vi "C867_Init.vi"(8 "error in":errorcluster caption="entrée d'erreur") -> (0 "error out":errorcluster caption="sortie d'erreur", 3 "ID":i32 caption="Numérique")   [LabVIEW 2026]
uses:
  Controls/TypeDef_FGV.ctl
  C867-VIs/Low Level/PI_GCS2_DLL_x64.dll
panel:
  in  "nBaudRate":i32=115200
  in  "nPortNr":i32=15
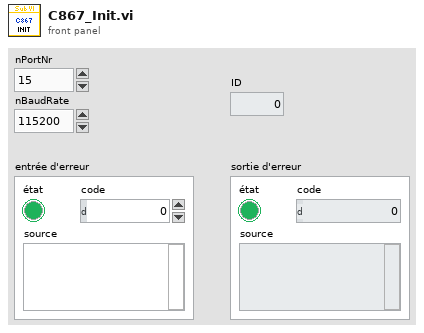
[diagram p1: front panel]
types:
  T1 = typedef "TypeDef_FGV.ctl" = enum16{"Initialize", "Write", "Read"}
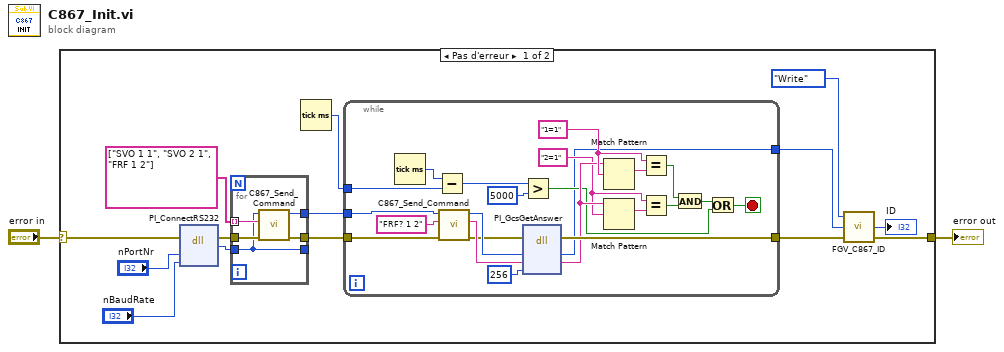
[diagram p0: block diagram]
diagram:
  n1 = case shown="Pas d'erreur" "error in" {
    selector: "error in" -> [w16 w45]
    tunnel: [w8 w45] -> w1
    frame No Error {
      n2 = dll-call lib="D:/SEBASTIEN/GitHub/LABVIEW-Useful-codes/Device_control/PC-C867-IO Control/v0.2/SubVI/PI-C867/C867-VIs/Low Level/PI_GCS2_DLL_x64.dll" fn="PI_ConnectRS232"(error in=w16, "nPortNr"="nPortNr", "nBaudRate"="nBaudRate") -> (error out=w5:errorcluster, "ID"=w6:i32)  [unwired: 4 in, 1 out]
      n3 = for {
        tunnel: string[] ["SVO 1 1", "SVO 2 1", "FRF 1 2"] -> [w18] mode=indexing
        tunnel: w5 -> [w21]
        tunnel: [w20] -> w11
        tunnel: [w17] -> _
        tunnel: [w19] -> w10
        tunnel: w6 -> [w17]
        n4 = call "C867_Send_Command.vi"("entrée d'erreur (pas d'erreur)"=w21, "szCommand"=w18, "ID en entrée"=w17) -> ("sortie d'erreur"=w20:errorcluster, "ID en sortie"=w19:i32)  [unwired: 5 in, 2 out]
      }
      n5 = Tick Count (ms)() -> (millisecond timer value=w13:u32)
      n6 = while {
        tunnel: w11 -> [w27]
        tunnel: w10 -> [w25]
        tunnel: [w44] -> w4
        tunnel: w13 -> [w41]
        tunnel: [w28] -> w3
        stop <- w31 stop-if-true
        w34 = "2=1" ("chaîne recherchée")
        w38 = "1=1" ("chaîne recherchée")
        n7 = Tick Count (ms)() -> (millisecond timer value=w42:u32)
        n8 = Subtract(x=w42, y=w41) -> (x-y=w40:u32)
        n9 = call "C867_Send_Command.vi"("entrée d'erreur (pas d'erreur)"=w27, "szCommand"="FRF? 1 2", "ID en entrée"=w25) -> ("sortie d'erreur"=w22:errorcluster, "szCommand out"=w24:string, "ID en sortie"=w23:i32)  [unwired: 5 in, 1 out]
        n10 = Greater?(x=w40, y=u32 5000) -> (0:w32:bool)
        n11 = dll-call lib="D:/SEBASTIEN/GitHub/LABVIEW-Useful-codes/Device_control/PC-C867-IO Control/v0.2/SubVI/PI-C867/C867-VIs/Low Level/PI_GCS2_DLL_x64.dll" fn="PI_GcsGetAnswer"(error in=w22, "ID"=w23, "buffer"=w24, "buffersize"=256) -> (error out=w44:errorcluster, "ID"=w28:i32, "buffer"=w36:string)  [unwired: 4 in, 1 out]
        n12 = Match Pattern(string=w36, regular expression=w38) -> (match substring=w37:string)  [unwired: 1 in, 3 out]
        n13 = Match Pattern(string=w36, regular expression=w34) -> (match substring=w35:string)  [unwired: 1 in, 3 out]
        n14 = Equal?(x=w38, y=w37) -> (x = y?=w30:bool)
        n15 = Equal?(x=w34, y=w35) -> (x = y?=w29:bool)
        n16 = And(x=w30, y=w29) -> (x .and. y?=w33:bool)
        n17 = Or(x=w33, y=w32) -> (x .or. y?=w31:bool)
      }
      n18 = call "FGV_C867_ID.vi"("error in"=w4, "ID"=w3, "Action"=TypeDef_FGV."Write") -> ("error out"=w8:errorcluster, "ID"=→"ID":i32)  [unwired: 1 in]
    }
    frame Error {
    }
  }
  "error out" <- w1
